vi "first call.vi"(0 "current subState":T1) -> (1 "current subState out":T1, 2 "x != y?":bool)   [LabVIEW 2011]
uses:
  typedefs/subStates.ctl
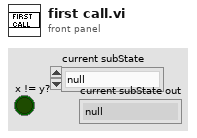
[diagram p1: front panel]
types:
  T1 = typedef "subStates.ctl" = enum16{"null", "wait", "driver control", "auto", "manual override", "hold position", "rotate", "end"}
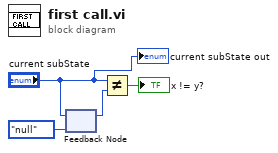
[diagram p0: block diagram]
diagram:
  n1 = feedback #1(subStates."null" ("subState out")) -> (w2:T1)
  n2 = feedback-in #1("current subState") -> ()
  n3 = Not Equal?(x="current subState", y=w2) -> (x != y?=→"x != y?":bool)
  "current subState out" <- "current subState"
